vi "robotkolkontrol2.vi"() -> ()   [LabVIEW 2016]
uses:
  <vilib>/LabVIEW Interface for Arduino/LabVIEW Interface for Arduino.lvlib
panel:
  out "Q2 2":dbl
  out "Q1 2":dbl
  in  "y  2":dbl
  in  "x  2":dbl
  in  "l2 2":dbl
  in  "l1 2":dbl
  out "Q2":dbl
  out "Q1":dbl
  in  "l2":dbl
  in  "l1":dbl
  in  "çalışma hızı":dbl
  in  "stop":bool
  in  "Number of Servos":u8=2
  in  "x":dbl
  in  "y":dbl
  in  "motor1":dbl(knob) scale=0.0..180.0
  out "Servo 0":dbl(knob) scale=0.0..180.0
  out "Servo 1":dbl(knob) scale=0.0..150.0
  in  "motor 2":dbl(knob) scale=0.0..90.0
  out "Servo 2":dbl(knob) scale=0.0..90.0
  in  "açma-kapama":dbl(knob) scale=0.0..120.0
  in  "otomatik(aç)-manuel(kapa)":bool
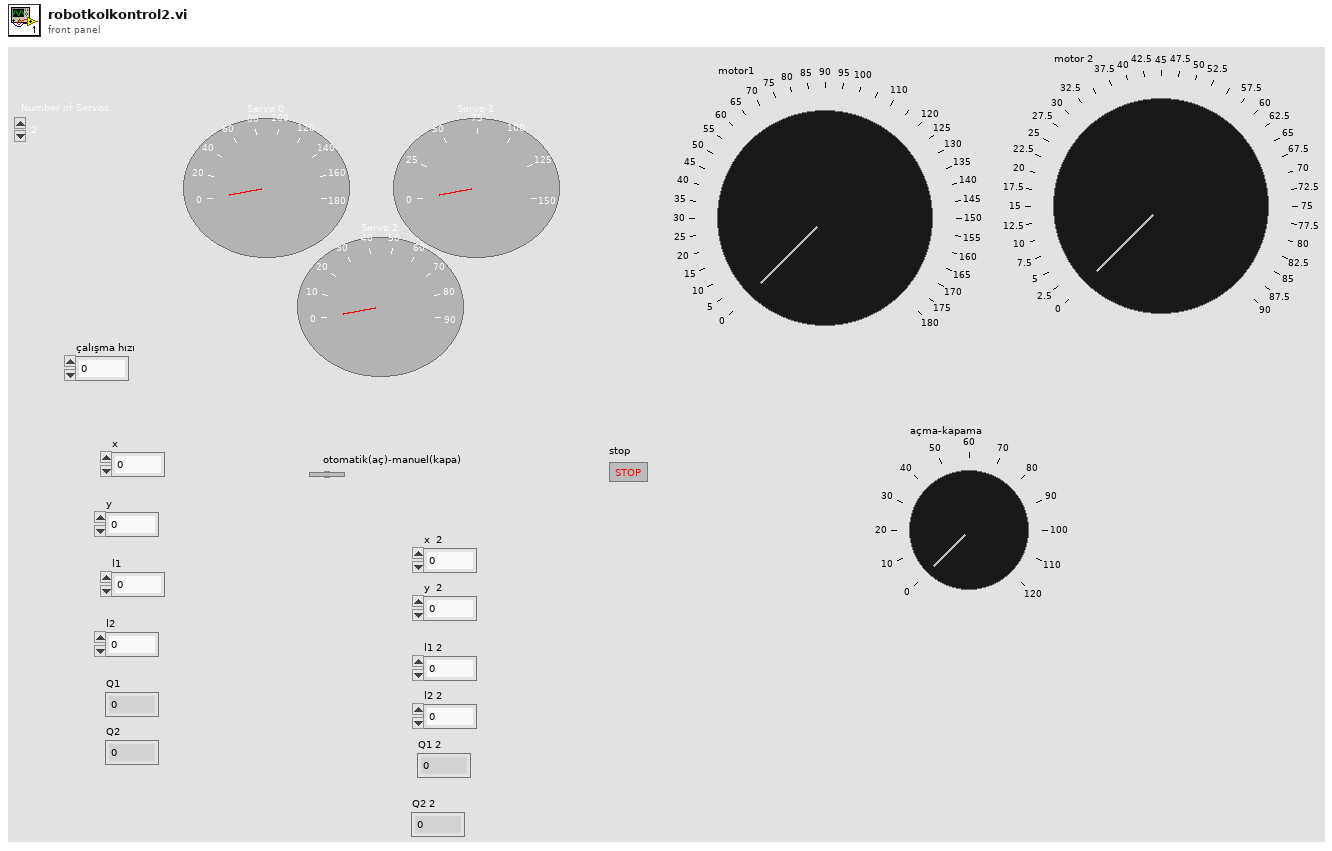
[diagram p1: front panel]
types:
  T1 = typedef "LabVIEW Interface for Arduino.lvlib/Arduino Resource.ctl" = cluster{"VISA resource":refnum<visa-resource-name>, "Board Type":T2, "Connection Type":enum8{"USB / Serial"}, "Bytes Per Packet (15)":u8}
  T2 = typedef "LabVIEW Interface for Arduino.lvlib/Board Type.ctl" = enum16{"Uno", "Dimuelanove w/Atmega 328", "Mega 2560"}
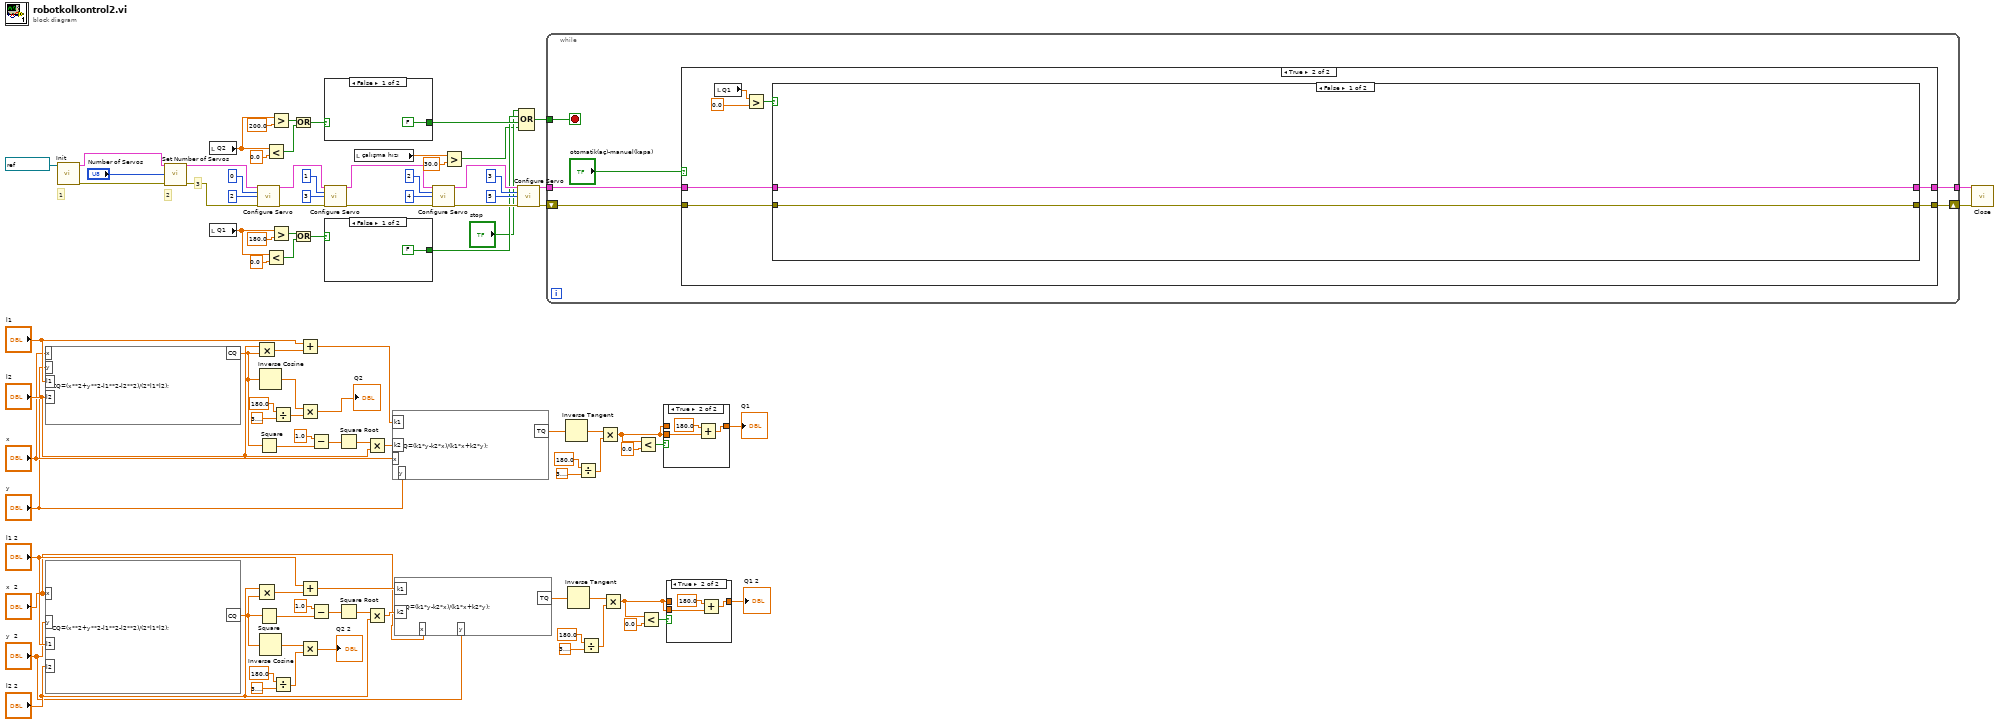
[diagram p0: block diagram]
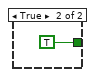
[diagram p4: hidden frame]
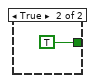
[diagram p5: hidden frame]
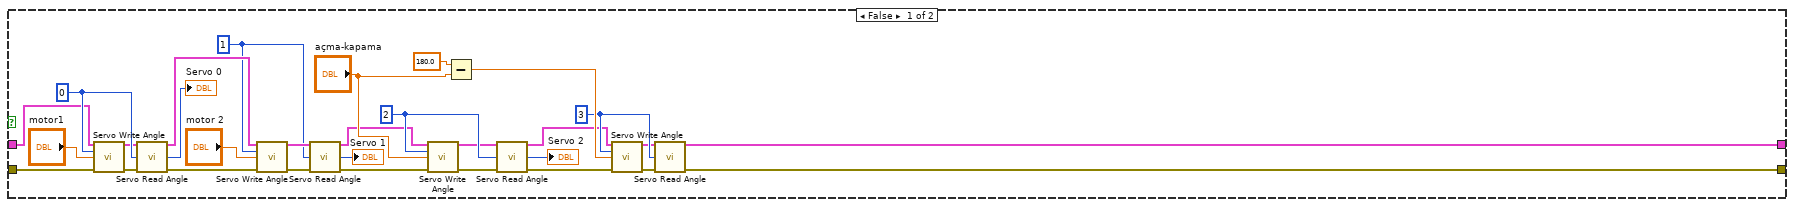
[diagram p6: hidden frame]
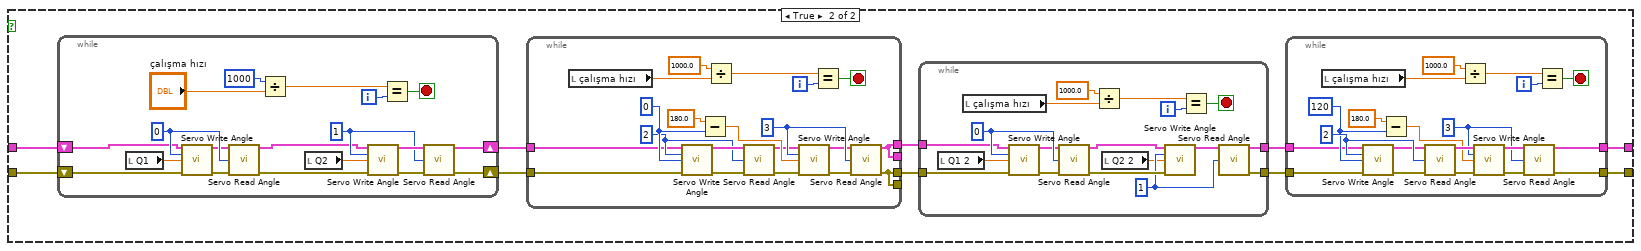
[diagram p7: hidden frame]
diagram:
  # "3"
  # "2"
  # "1"
  n1 = formula code="CQ=(x**2+y**2-l1**2-l2**2)/(2*l1*l2);"("x"="x", "y"="y", "l1"="l1", "l2"="l2") -> ("CQ"=w37:dbl)
  n2 = formula code="CQ=(x**2+y**2-l1**2-l2**2)/(2*l1*l2);"("x"="x  2", "y"="y  2", "l1"="l1 2", "l2"="l2 2") -> ("CQ"=w21:dbl)
  n3 = call <vilib>:"Init.vi"("VISA resource"=refnum<visa-resource-name> "COM3") -> ("Arduino Resource"=w95:T1, "error out"=w94:errorcluster)  [unwired: 17 in]
  n4 = call <vilib>:"Set Number of Servos.vi"("Arduino Resource"=w95, "Number Of Servos (1)"="Number of Servos", "error in"=w94) -> ("Arduino Resource"=w92:T1, "error out"=w91:errorcluster)  [unwired: 11 in]
  n5 = local read "Q2"() -> (w63:dbl)
  n6 = local read "Q1"() -> (w69:dbl)
  n7 = Multiply(x="l2", y=w37) -> (x*y=w48:dbl)
  n8 = Multiply(x="l2 2", y=w21) -> (x*y=w32:dbl)
  n9 = call <vilib>:"Configure Servo.vi"("Arduino Resource"=w92, "Servo Number (0)"=u8 0 ("Servo Number"), "DIO Pin (2)"=u8 2 ("Servo Number"), "error in"=w91) -> ("Arduino Resource"=w90:T1, "error out"=w89:errorcluster)  [unwired: 10 in]
  n10 = Square(x=w37) -> (x^2=w52:dbl)
  n11 = Square(x=w21) -> (x^2=w36:dbl)
  n12 = Inverse Cosine(1:w37) -> (0:w39:dbl)
  n13 = Inverse Cosine(1:w21) -> (0:w23:dbl)
  n14 = Less?(x=w63, y=0.0) -> (x < y?=w65:bool)
  n15 = Less?(x=w69, y=0.0) -> (x < y?=w71:bool)
  n16 = Greater?(x=w63, y=200.0) -> (0:w61:bool)
  n17 = Greater?(x=w69, y=180.0) -> (0:w68:bool)
  n18 = Divide(x=180.0, y=3.141592653589793) -> (x/y=w38:dbl)
  n19 = Divide(x=180.0, y=3.141592653589793) -> (x/y=w22:dbl)
  n20 = Or(x=w61, y=w65) -> (x .or. y?=w62:bool)
  n21 = Or(x=w68, y=w71) -> (x .or. y?=w67:bool)
  n22 = Add(x="l1", y=w48) -> (x+y=w19:dbl)
  n23 = Multiply(x=w39, y=w38) -> (x*y=→"Q2":dbl)
  n24 = Add(x="l1 2", y=w32) -> (x+y=w14:dbl)
  n25 = Multiply(x=w23, y=w22) -> (x*y=→"Q2 2":dbl)
  n26 = Subtract(x=1.0, y=w52) -> (x-y=w50:dbl)
  n27 = Subtract(x=1.0, y=w36) -> (x-y=w34:dbl)
  n28 = case shown="False" w62 {
    tunnel: [FALSE TRUE] -> w60
    frame False {
    }
    frame True {
    }
  }
  n29 = call <vilib>:"Configure Servo.vi"("Arduino Resource"=w90, "Servo Number (0)"=u8 1 ("Servo Number"), "DIO Pin (2)"=u8 3 ("Servo Number"), "error in"=w89) -> ("Arduino Resource"=w83:T1, "error out"=w82:errorcluster)  [unwired: 10 in]
  n30 = case shown="False" w67 {
    tunnel: [FALSE TRUE] -> w58
    frame False {
    }
    frame True {
    }
  }
  n31 = Square Root(x=w50) -> (sqrt(x)=w47:dbl)
  n32 = Square Root(x=w34) -> (sqrt(x)=w31:dbl)
  n33 = local read "çalışma hızı"() -> (w53:dbl)
  n34 = Multiply(x=w47, y="l2") -> (x*y=w20:dbl)
  n35 = Multiply(x=w31, y="l2 2") -> (x*y=w13:dbl)
  n36 = formula code="TQ=(k1*y-k2*x)/(k1*x+k2*y);"("k1"=w19, "k2"=w20, "x"="x", "y"="y") -> ("TQ"=w18:dbl)
  n37 = formula code="TQ=(k1*y-k2*x)/(k1*x+k2*y);"("k1"=w14, "k2"=w13, "x"="x  2", "y"="y  2") -> ("TQ"=w17:dbl)
  n38 = call <vilib>:"Configure Servo.vi"("Arduino Resource"=w83, "Servo Number (0)"=u8 2, "DIO Pin (2)"=u8 4, "error in"=w82) -> ("Arduino Resource"=w79:T1, "error out"=w78:errorcluster)  [unwired: 10 in]
  n39 = Greater?(x=w53, y=30.0) -> (0:w55:bool)
  n40 = call <vilib>:"Configure Servo.vi"("Arduino Resource"=w79, "Servo Number (0)"=u8 3, "DIO Pin (2)"=u8 5, "error in"=w78) -> ("Arduino Resource"=w77:T1, "error out"=w76:errorcluster)  [unwired: 10 in]
  n41 = Compound Arithmetic op=OR("stop", w58, w60, w55) -> (w56:bool)
  n42 = while {
    tunnel: w77 -> [w104]
    shift-right: [w101] -> w73
    shift-left: w76 -> [w103]
    tunnel: [w102] -> w72
    tunnel: w56 -> [w100]
    stop <- w100 stop-if-true
    n43 = case shown="True" "otomatik(aç)-manuel(kapa)" {
      tunnel: w104 -> [w131 w142]
      tunnel: w103 -> [w130 w141]
      tunnel: [w109 w140] -> w102
      tunnel: [w110 w139] -> w101
      frame False {
        w120 = u8 3 ("Servo Number")
        w115 = u8 2 ("Servo Number")
        w108 = u8 1 ("Servo Number")
        w135 = u8 0 ("Servo Number")
        n44 = call <vilib>:"Servo Write Angle.vi"("Arduino Resource"=w131, "Servo Number"=w135, "Angle (Degrees)"="motor1", "error in"=w130) -> ("Arduino Resource"=w133:T1, "error out"=w134:errorcluster)  [unwired: 10 in]
        n45 = call <vilib>:"Servo Read Angle.vi"("Arduino Resource"=w133, "Servo Number"=w135, "error in"=w134) -> ("Arduino Resource"=w125:T1, "Angle (Degrees)"=→"Servo 0":u8, "error out"=w124:errorcluster)  [unwired: 10 in]
        n46 = call <vilib>:"Servo Write Angle.vi"("Arduino Resource"=w125, "Servo Number"=w108, "Angle (Degrees)"="motor 2", "error in"=w124) -> ("Arduino Resource"=w128:T1, "error out"=w127:errorcluster)  [unwired: 10 in]
        n47 = call <vilib>:"Servo Read Angle.vi"("Arduino Resource"=w128, "Servo Number"=w108, "error in"=w127) -> ("Arduino Resource"=w107:T1, "Angle (Degrees)"=→"Servo 1":u8, "error out"=w106:errorcluster)  [unwired: 10 in]
        n48 = call <vilib>:"Servo Write Angle.vi"("Arduino Resource"=w107, "Servo Number"=w115, "Angle (Degrees)"="açma-kapama", "error in"=w106) -> ("Arduino Resource"=w113:T1, "error out"=w114:errorcluster)  [unwired: 10 in]
        n49 = Subtract(x=180.0, y="açma-kapama") -> (x-y=w121:dbl)
        n50 = call <vilib>:"Servo Read Angle.vi"("Arduino Resource"=w113, "Servo Number"=w115, "error in"=w114) -> ("Arduino Resource"=w116:T1, "Angle (Degrees)"=→"Servo 2":u8, "error out"=w117:errorcluster)  [unwired: 10 in]
        n51 = call <vilib>:"Servo Write Angle.vi"("Arduino Resource"=w116, "Servo Number"=w120, "Angle (Degrees)"=w121, "error in"=w117) -> ("Arduino Resource"=w118:T1, "error out"=w119:errorcluster)  [unwired: 10 in]
        n52 = call <vilib>:"Servo Read Angle.vi"("Arduino Resource"=w118, "Servo Number"=w120, "error in"=w119) -> ("Arduino Resource"=w109:T1, "error out"=w110:errorcluster)  [unwired: 10 in, 1 out]
      }
      frame True {
        n53 = local read "Q1"() -> (w137:dbl)
        n54 = Greater?(x=w137, y=0.0) -> (0:w138:bool)
        n55 = case shown="False" w138 {
          tunnel: w142 -> [w144 w154]
          tunnel: w141 -> [w143 w153]
          tunnel: [w144 w152] -> w140
          tunnel: [w143 w151] -> w139
          frame False {
          }
          frame True {
            n56 = while {
              shift-right: [w206] -> w148
              shift-left: w154 -> [w202]
              shift-right: [w205] -> w147
              shift-left: w153 -> [w201]
              i -> [w200]
              stop <- w207 stop-if-true
              w208 = u8 1 ("Servo Number")
              w213 = u8 0 ("Servo Number")
              n57 = local read "Q1"() -> (w196:dbl)
              n58 = call <vilib>:"Servo Write Angle.vi"("Arduino Resource"=w202, "Servo Number"=w213, "Angle (Degrees)"=w196, "error in"=w201) -> ("Arduino Resource"=w211:T1, "error out"=w212:errorcluster)  [unwired: 10 in]
              n59 = call <vilib>:"Servo Read Angle.vi"("Arduino Resource"=w211, "Servo Number"=w213, "error in"=w212) -> ("Arduino Resource"=w204:T1, "error out"=w203:errorcluster)  [unwired: 10 in, 1 out]
              n60 = Divide(x=1000, y="çalışma hızı") -> (x/y=w197:dbl)
              n61 = local read "Q2"() -> (w195:dbl)
              n62 = call <vilib>:"Servo Write Angle.vi"("Arduino Resource"=w204, "Servo Number"=w208, "Angle (Degrees)"=w195, "error in"=w203) -> ("Arduino Resource"=w210:T1, "error out"=w209:errorcluster)  [unwired: 10 in]
              n63 = Equal?(x=w197, y=w200) -> (x = y?=w207:bool)
              n64 = call <vilib>:"Servo Read Angle.vi"("Arduino Resource"=w210, "Servo Number"=w208, "error in"=w209) -> ("Arduino Resource"=w206:T1, "error out"=w205:errorcluster)  [unwired: 10 in, 1 out]
            }
            n65 = while {
              tunnel: [w159] -> _
              tunnel: [w158] -> _
              tunnel: w148 -> [w161]
              tunnel: w147 -> [w160]
              tunnel: [w159] -> w146
              tunnel: [w158] -> w145
              i -> [w163]
              stop <- w162 stop-if-true
              w166 = 0
              w165 = u8 2 ("Servo Number")
              w170 = u8 3 ("Servo Number")
              n66 = local read "çalışma hızı"() -> (w157:dbl)
              n67 = call <vilib>:"Servo Write Angle.vi"("Arduino Resource"=w161, "Servo Number"=w165, "Angle (Degrees)"=w166, "error in"=w160) -> ("Arduino Resource"=w169:T1, "error out"=w171:errorcluster)  [unwired: 10 in]
              n68 = Subtract(x=180.0, y=w166) -> (x-y=w174:dbl)
              n69 = Divide(x=1000.0, y=w157) -> (x/y=w156:dbl)
              n70 = call <vilib>:"Servo Read Angle.vi"("Arduino Resource"=w169, "Servo Number"=w165, "error in"=w171) -> ("Arduino Resource"=w168:T1, "error out"=w172:errorcluster)  [unwired: 10 in, 1 out]
              n71 = call <vilib>:"Servo Write Angle.vi"("Arduino Resource"=w168, "Servo Number"=w170, "Angle (Degrees)"=w174, "error in"=w172) -> ("Arduino Resource"=w167:T1, "error out"=w173:errorcluster)  [unwired: 10 in]
              n72 = Equal?(x=w156, y=w163) -> (x = y?=w162:bool)
              n73 = call <vilib>:"Servo Read Angle.vi"("Arduino Resource"=w167, "Servo Number"=w170, "error in"=w173) -> ("Arduino Resource"=w159:T1, "error out"=w158:errorcluster)  [unwired: 10 in, 1 out]
            }
            n74 = while {
              tunnel: [w222] -> w150
              tunnel: [w221] -> w149
              tunnel: w146 -> [w220]
              tunnel: w145 -> [w219]
              i -> [w227]
              stop <- w228 stop-if-true
              w223 = u8 1 ("Servo Number")
              w231 = u8 0 ("Servo Number")
              n75 = local read "Q1 2"() -> (w215:dbl)
              n76 = local read "çalışma hızı"() -> (w218:dbl)
              n77 = call <vilib>:"Servo Write Angle.vi"("Arduino Resource"=w220, "Servo Number"=w231, "Angle (Degrees)"=w215, "error in"=w219) -> ("Arduino Resource"=w229:T1, "error out"=w230:errorcluster)  [unwired: 10 in]
              n78 = call <vilib>:"Servo Read Angle.vi"("Arduino Resource"=w229, "Servo Number"=w231, "error in"=w230) -> ("Arduino Resource"=w225:T1, "error out"=w224:errorcluster)  [unwired: 10 in, 1 out]
              n79 = Divide(x=1000.0, y=w218) -> (x/y=w216:dbl)
              n80 = local read "Q2 2"() -> (w214:dbl)
              n81 = call <vilib>:"Servo Write Angle.vi"("Arduino Resource"=w225, "Servo Number"=w223, "Angle (Degrees)"=w214, "error in"=w224) -> ("Arduino Resource"=w226:T1)  [unwired: 10 in, 1 out]
              n82 = Equal?(x=w216, y=w227) -> (x = y?=w228:bool)
              n83 = call <vilib>:"Servo Read Angle.vi"("Arduino Resource"=w226, "Servo Number"=w223) -> ("Arduino Resource"=w222:T1, "error out"=w221:errorcluster)  [unwired: 11 in, 1 out]
            }
            n84 = while {
              tunnel: [w182] -> w152
              tunnel: [w181] -> w151
              tunnel: w150 -> [w179]
              tunnel: w149 -> [w178]
              i -> [w183]
              stop <- w184 stop-if-true
              w180 = 120
              w189 = u8 3 ("Servo Number")
              w191 = u8 2 ("Servo Number")
              n85 = local read "çalışma hızı"() -> (w177:dbl)
              n86 = call <vilib>:"Servo Write Angle.vi"("Arduino Resource"=w179, "Servo Number"=w191, "Angle (Degrees)"=w180, "error in"=w178) -> ("Arduino Resource"=w190:T1, "error out"=w188:errorcluster)  [unwired: 10 in]
              n87 = Subtract(x=180.0, y=w180) -> (x-y=w185:dbl)
              n88 = call <vilib>:"Servo Read Angle.vi"("Arduino Resource"=w190, "Servo Number"=w191, "error in"=w188) -> ("Arduino Resource"=w192:T1, "error out"=w187:errorcluster)  [unwired: 10 in, 1 out]
              n89 = Divide(x=1000.0, y=w177) -> (x/y=w175:dbl)
              n90 = call <vilib>:"Servo Write Angle.vi"("Arduino Resource"=w192, "Servo Number"=w189, "Angle (Degrees)"=w185, "error in"=w187) -> ("Arduino Resource"=w193:T1, "error out"=w186:errorcluster)  [unwired: 10 in]
              n91 = call <vilib>:"Servo Read Angle.vi"("Arduino Resource"=w193, "Servo Number"=w189, "error in"=w186) -> ("Arduino Resource"=w182:T1, "error out"=w181:errorcluster)  [unwired: 10 in, 1 out]
              n92 = Equal?(x=w175, y=w183) -> (x = y?=w184:bool)
            }
          }
        }
      }
    }
  }
  n93 = Inverse Tangent(1:w18) -> (0:w45:dbl)
  n94 = Inverse Tangent(1:w17) -> (0:w29:dbl)
  n95 = Divide(x=180.0, y=3.141592653589793) -> (x/y=w44:dbl)
  n96 = Divide(x=180.0, y=3.141592653589793) -> (x/y=w28:dbl)
  n97 = Multiply(x=w45, y=w44) -> (x*y=w7:dbl)
  n98 = Multiply(x=w29, y=w28) -> (x*y=w4:dbl)
  n99 = Less?(x=w7, y=0.0) -> (x < y?=w10:bool)
  n100 = Less?(x=w4, y=0.0) -> (x < y?=w6:bool)
  n101 = case shown="True" w10 {
    tunnel: [w232 w233] -> w8
    tunnel: w7 -> [_ w234]
    tunnel: w7 -> [w232 _]
    frame False {
    }
    frame True {
      n102 = Add(x=180.0, y=w234) -> (x+y=w233:dbl)
    }
  }
  "Q1" <- w8
  n103 = case shown="True" w6 {
    tunnel: [w236 w237] -> w3
    tunnel: w4 -> [_ w238]
    tunnel: w4 -> [w236 _]
    frame False {
    }
    frame True {
      n104 = Add(x=180.0, y=w238) -> (x+y=w237:dbl)
    }
  }
  "Q1 2" <- w3
  n105 = call <vilib>:"Close.vi"("Arduino Resource"=w72, "error in"=w73) -> ()  [unwired: 13 in, 1 out]
